vi "CustomConstructService.vi"(11 "MicronConfig":T1) -> (1 "MicronMessageQueue":refnum<queue>, 2 "MicronMessageUE":refnum<user-event>, 3 "MicronGRPC out":refnum<class "MicronGRPC.lvclass">)   [LabVIEW 2019, in "MicronGRPCGeneratedServer.lvlib"]
uses:
  MicronGRPCGeneratedServer.lvlib
  RPC Service/MicronGRPC/MicronGRPC.lvclass
  Base/Server/Message/MessageBase.lvclass
  Base/Server/Service/Typedefs/MicronConfig.ctl
  Base/Server/Service/ServiceBase.lvclass
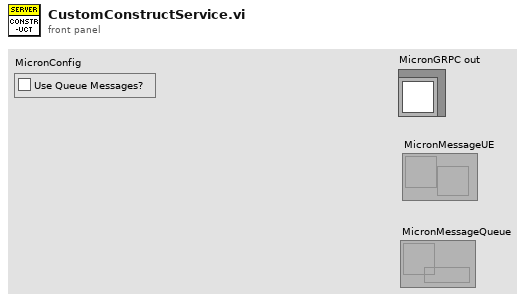
[diagram p1: front panel]
types:
  T1 = typedef "MicronServer.lvlib/ServiceBase.lvclass/MicronConfig.ctl" = cluster{"Use Queue Messages?":bool}
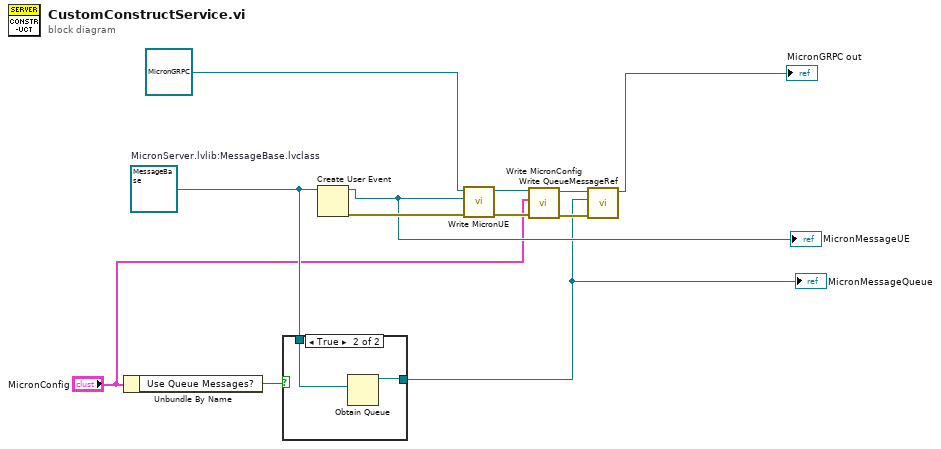
[diagram p0: block diagram]
diagram:
  w9 = refnum<class "MessageBase.lvclass"> refnum  # MicronServer.lvlib:MessageBase.lvclass
  n1 = Unbundle By Name("MicronConfig") -> ("Use Queue Messages?"=w8:bool)
  n2 = case shown="True" w8 {
    tunnel: w9 -> [_ w14]
    tunnel: [_ w13] -> w1
    frame False {
    }
    frame True {
      n3 = Obtain Queue(element data type=w14) -> (queue out=w13:refnum<queue>)  [unwired: 4 in, 2 out]
    }
  }
  "MicronMessageQueue" <- w1
  n4 = Create User Event(user event datatype=w9) -> (user event=w10:refnum<user-event>, error out=w12:errorcluster)  [unwired: 1 in]
  "MicronMessageUE" <- w10
  n5 = call-dynamic "Write MicronUE.vi"("error in (no error)"=w12, "MicronUE"=w10, "MicronGRPC in"=refnum<class "MicronGRPC.lvclass"> refnum ("MicronGRPCGeneratedServer.lvlib:MicronGRPC.lvclass")) -> ("error out"=w4:errorcluster, "MicronGRPC out"=w7:refnum<class "MicronGRPC.lvclass">)  [unwired: 7 in]
  n6 = call-dynamic "Write MicronConfig.vi"("error in (no error)"=w4, "MicronConfig"="MicronConfig", "MicronGRPC in"=w7) -> ("error out"=w3:errorcluster, "MicronGRPC out"=w6:refnum<class "MicronGRPC.lvclass">)  [unwired: 7 in]
  n7 = call-dynamic "Write QueueMessageRef.vi"("error in (no error)"=w3, "QueueMessageRef"=w1, "MicronGRPC in"=w6) -> ("MicronGRPC out"=→"MicronGRPC out":refnum<class "MicronGRPC.lvclass">)  [unwired: 7 in, 1 out]
